vi "LoadConfigFile.vi"(0 "error in (no error)":errorcluster) -> (20 "error out":errorcluster, 21 "IP":string caption="Robot IP Address", 22 "Licensee":string, 23 "Key":string)   [LabVIEW 2018]
uses:
  <vilib>/Utility/config.llb/NI_LVConfig.lvlib
  <vilib>/Utility/config.llb/Read Key (String).vi
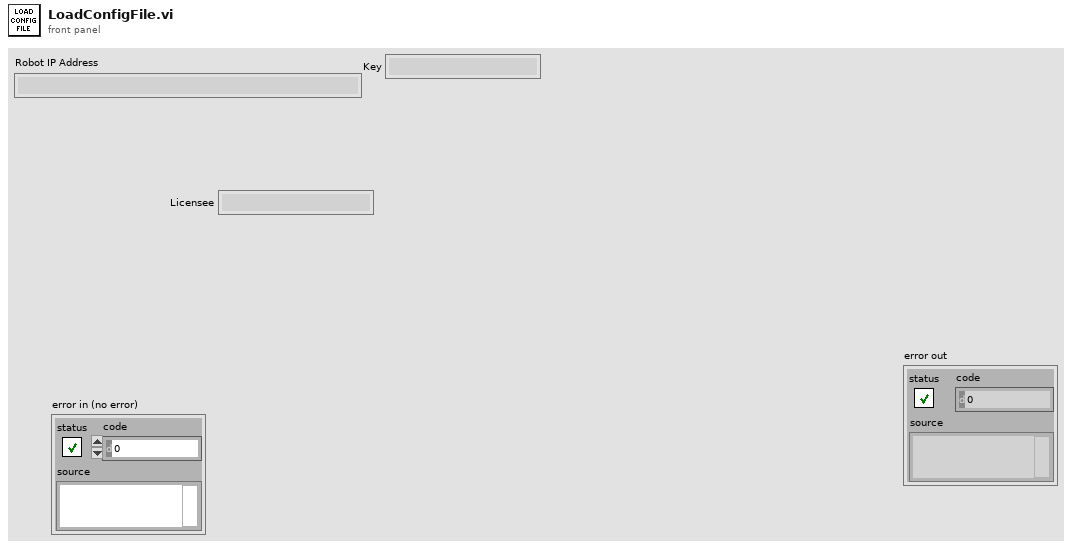
[diagram p1: front panel]
types:
  T1 = typedef "NI_LVConfig.lvlib/Config Data RefNum.ctl" = refnum<k1>
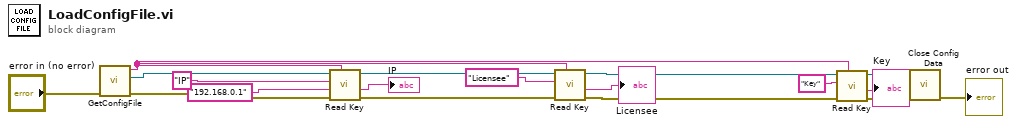
[diagram p0: block diagram]
diagram:
  n1 = call "GetConfigFile.vi"("error in (no error)"="error in (no error)") -> ("error out"=w17:errorcluster, "refnum"=w16:T1, "section"=w8:string)  [unwired: 8 in]
  n2 = call-poly <vilib>:"Read Key.vi"("section"=w8, "error in (no error)"=w17, "default value"="192.168.0.1", "key"="IP", "refnum"=w16) -> ("error out"=w2:errorcluster, "value"=→"IP":string, "refnum out"=w1:T1)  [unwired: 3 in, 1 out]
  n3 = call-poly <vilib>:"Read Key.vi"("section"=w8, "error in (no error)"=w2, "key"="Licensee", "refnum"=w1) -> ("error out"=w11:errorcluster, "value"=→"Licensee":string, "refnum out"=w12:T1)  [unwired: 4 in, 1 out]
  n4 = call-poly <vilib>:"Read Key.vi"("section"=w8, "error in (no error)"=w11, "key"="Key", "refnum"=w12) -> ("error out"=w10:errorcluster, "value"=→"Key":string, "refnum out"=w13:T1)  [unwired: 4 in, 1 out]
  n5 = call <vilib>:"Close Config Data.vi"("error in (no error)"=w10, "refnum"=w13) -> ("error out"=→"error out":errorcluster)  [unwired: 8 in, 1 out]
